vi "R30.vi"() -> ()   [LabVIEW 2016, in "beamline sections.lvlib" / "R30  library.lvlib"]
uses:
  R30/R30  library.lvlib
  save load/saveloadprev.ctl
  controls/Faraday cup states.ctl
  low energy end/Low energy end/Low energy end llb.lvlib
  Transmission/transmission.lvlib
  High energy end/High energy llb.lvlib
  save load/SaveLoad.lvlib
panel:
  in  "Tab Control":T1(tab)
  in  "Cluster 2":T2
  out "R30 steer +X":dbl
  out "R30 steer -X":dbl
  out "R30 steer +Y":dbl
  out "R30 steer -Y":dbl
  out "R30 steer +X Set":dbl
  out "R30 steer -X Set":dbl
  out "R30 steer +Y Set":dbl
  out "R30 steer -Y Set":dbl
  in  "stop":bool
  out "R30 Mag Y-steerer I read":dbl format="%#_3g"
  out "Mag Y-steerer range":bool=TRUE
  out "ESA range":bool=TRUE
  out "ESA V Read":dbl min=0.0 max=200.0
  in  "ESA":dbl(slide) min=0.0 max=60.0 scale=0.0..75.0
  in  "R30 Y steerer":dbl(slide) min=-10.0 max=10.0 scale=-10.0..10.0
  in  "R30 Quad A":dbl(slide) min=0.0 max=2.0 step=0.01 scale=0.0..2.0
  in  "R30 X steerer":dbl(slide) min=-10.0 max=10.0 scale=-10.0..10.0
  in  "R30 Quad B":dbl(slide) min=0.0 max=2.0 step=0.01 scale=0.0..2.0
  out "R30 Quad A I read":dbl min=0.0 max=200.0 format="%#_3g"
  out "R30 Quad B I read":dbl min=0.0 max=200.0 format="%#_3g"
  out "R30 quad Range":bool=TRUE
  out "R30 Steerer X Read":dbl format="%#_5g"
  out "R30 Steerer Y Read":dbl format="%#_4g"
  out "R30 Steerer range":bool=TRUE
  in  "Mag Y steerer":dbl(slide) min=-3.0 max=3.0 scale=-3.0..3.0
  out "R30 Mag Y-steerer V read":dbl
  out "R30 Detector FC status":T3
  in  "R30 temp file":path=path "D:/Main Tune Parameters/Temp Configs/R30.txt"
  out "SV error":errorcluster
  out "SaveLoad error":errorcluster
  out "R30-1-RT Error":errorcluster
  out "R30-1-FPGA Error":errorcluster
  # "R30"
  # "R30 Steerer Plate Voltages"
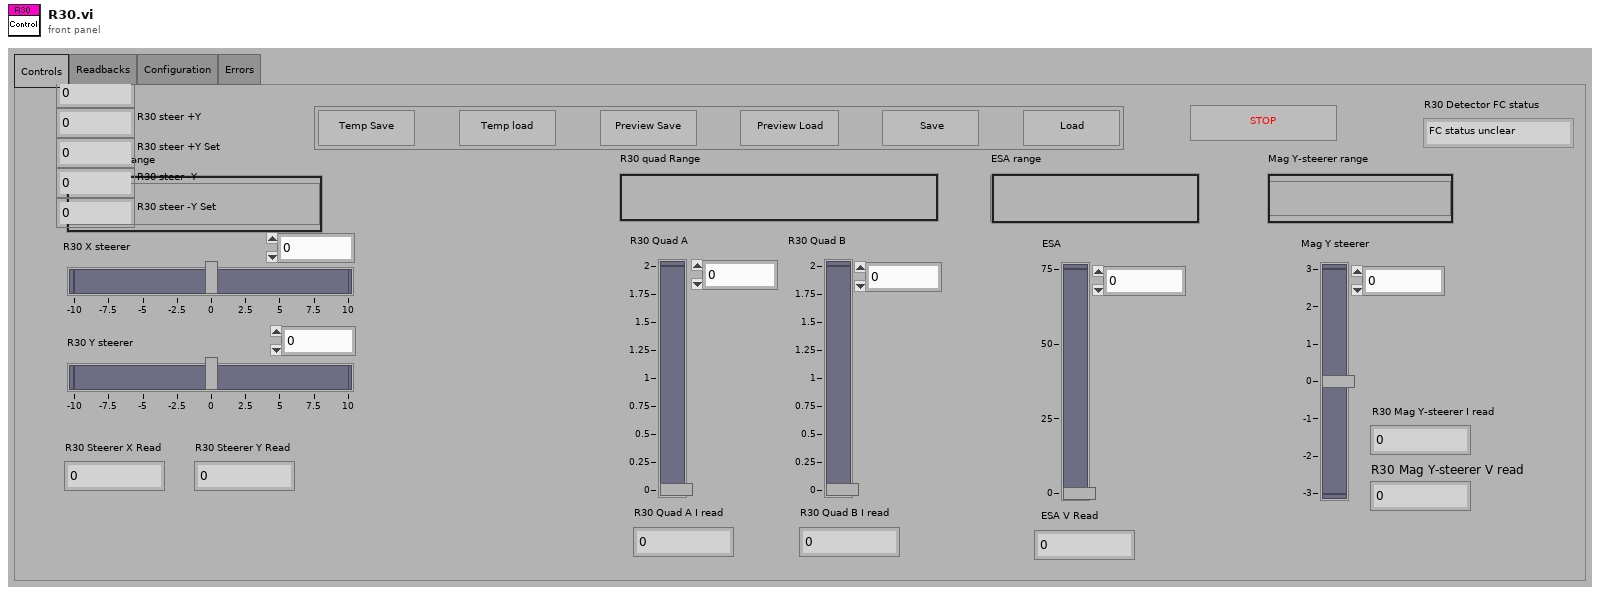
[diagram p1: front panel]
types:
  T1 = enum32{"Controls", "Readbacks", "Configuration", "Errors"}
  T2 = typedef "saveloadprev.ctl" = cluster{"Temp Save":bool, "Temp Load":bool, "Save":bool, "Load":bool, "Preview Save":bool, "Preview Load":bool}
  T3 = typedef "Faraday cup states.ctl" = enum16{"FC status unclear", "FC in", "FC out"}
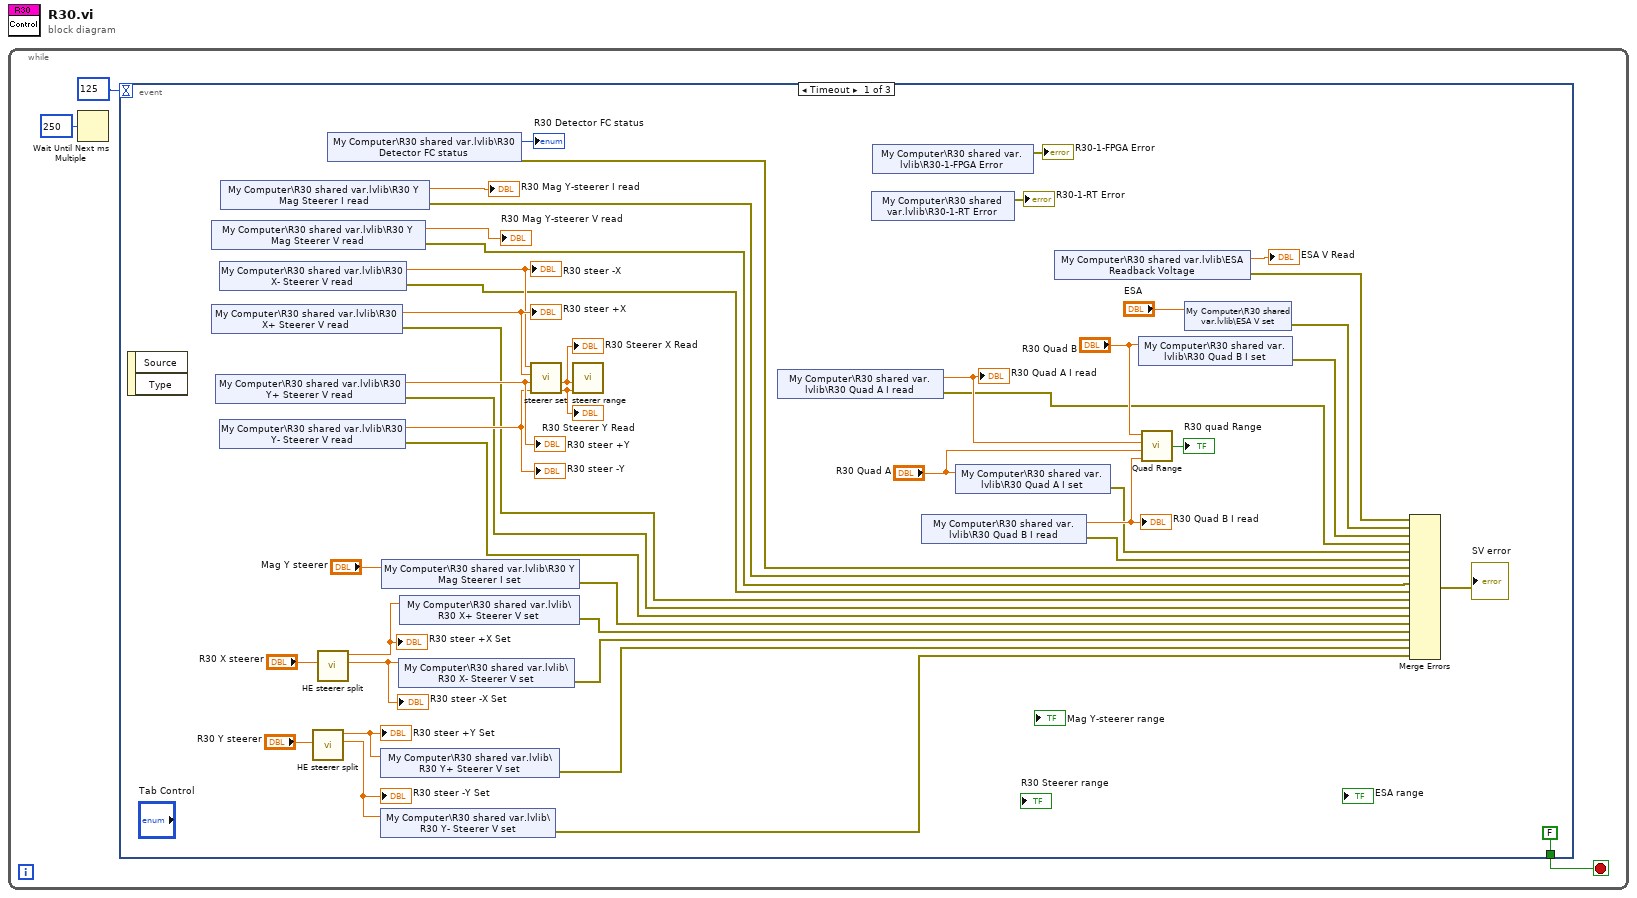
[diagram p0: block diagram]
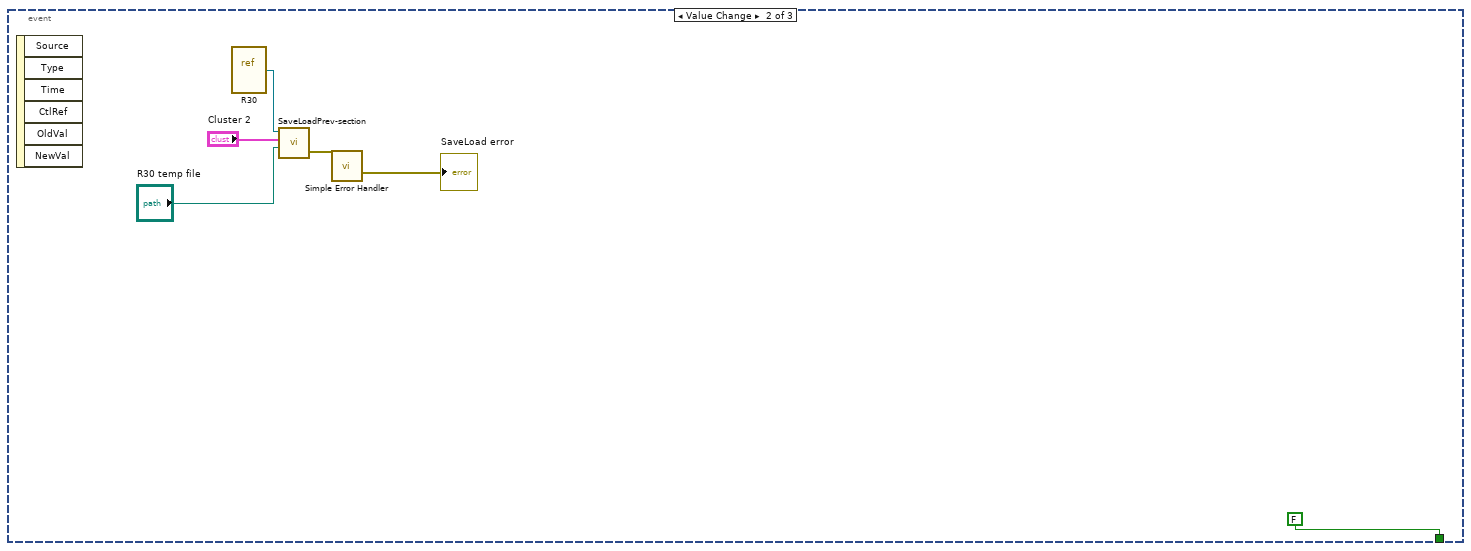
[diagram p2: hidden frame]
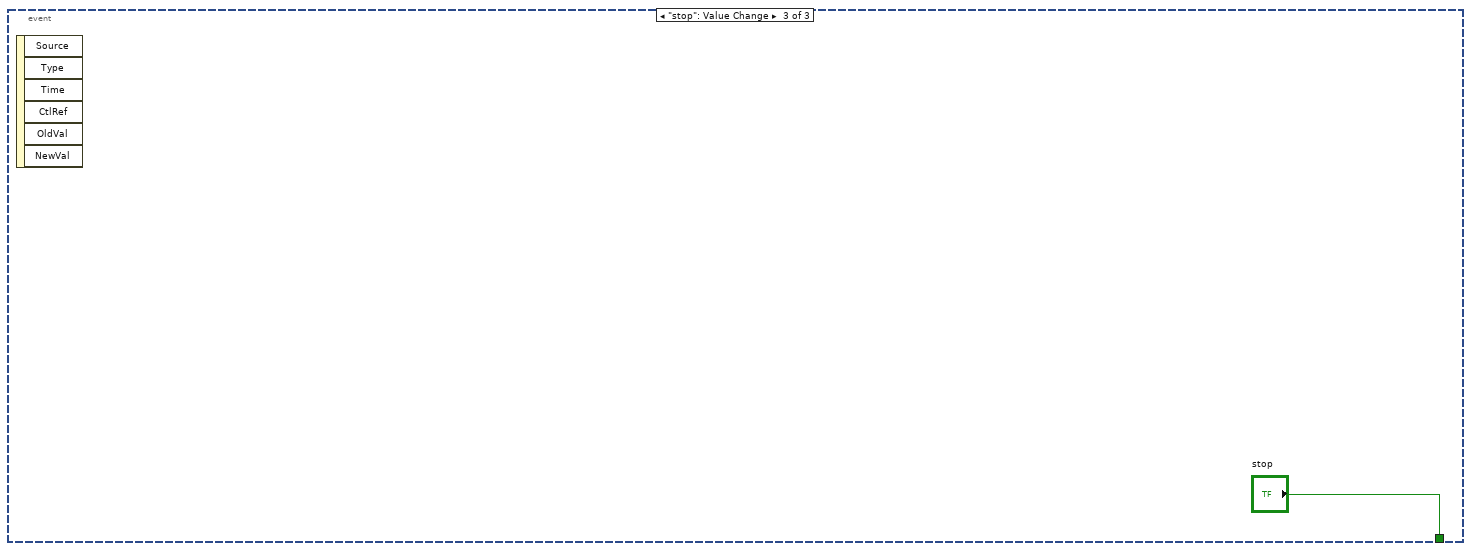
[diagram p3: hidden frame]
diagram:
  n1 = while {
    stop <- w1 stop-if-true
    n2 = Wait Until Next ms Multiple(millisecond multiple=u32 250) -> ()  [unwired: 1 out]
    n3 = event shown="[0] Timeout" {
      selector: _ -> [_ _ _]
      dyn-events: _ -> [_ _ _]
      timeout: 125 -> [_ _ _]
      tunnel: [FALSE ("stop") FALSE ("stop") "stop"] -> w1
      event Timeout {
        n4 = event-data() -> ()  [unwired: 1 in, 2 out]
        n5 = shared-variable "My Computer\\R30 shared var.lvlib\\R30 Y Mag Steerer V read"() -> (→"R30 Mag Y-steerer V read":dbl, error out=w6:errorcluster)  [unwired: 1 in]
        n6 = shared-variable "My Computer\\R30 shared var.lvlib\\R30 X+ Steerer V read"() -> (w43:dbl, error out=w20:errorcluster)  [unwired: 1 in]
        "R30 steer +X" <- w43
        n7 = shared-variable "My Computer\\R30 shared var.lvlib\\R30 Y+ Steerer V read"() -> (w47:dbl, error out=w21:errorcluster)  [unwired: 1 in]
        "R30 steer +Y" <- w47
        n8 = shared-variable "My Computer\\R30 shared var.lvlib\\R30 X- Steerer V read"() -> (w42:dbl, error out=w19:errorcluster)  [unwired: 1 in]
        "R30 steer -X" <- w42
        n9 = shared-variable "My Computer\\R30 shared var.lvlib\\R30 Y- Steerer V read"() -> (w46:dbl, error out=w22:errorcluster)  [unwired: 1 in]
        "R30 steer -Y" <- w46
        n10 = shared-variable "My Computer\\R30 shared var.lvlib\\R30 Y Mag Steerer I read"() -> (→"R30 Mag Y-steerer I read":dbl, error out=w18:errorcluster)  [unwired: 1 in]
        n11 = call "HE steerer split.vi"("Steerer in"="R30 Y steerer") -> ("Steerer +"=w36:dbl, "Steerer -"=w41:dbl)  [unwired: 7 out]
        "R30 steer +Y Set" <- w36
        "R30 steer -Y Set" <- w41
        n12 = call "HE steerer split.vi"("Steerer in"="R30 X steerer") -> ("Steerer +"=w39:dbl, "Steerer -"=w40:dbl)  [unwired: 7 out]
        "R30 steer +X Set" <- w39
        "R30 steer -X Set" <- w40
        n13 = shared-variable "My Computer\\R30 shared var.lvlib\\R30 Detector FC status"() -> (→"R30 Detector FC status":T3, error out=w17:errorcluster)  [unwired: 1 in]
        n14 = shared-variable "My Computer\\R30 shared var.lvlib\\R30 Y+ Steerer V set"(w36) -> (error out=w25:errorcluster)  [unwired: 1 in]
        n15 = shared-variable "My Computer\\R30 shared var.lvlib\\R30 Y- Steerer V set"(w41) -> (error out=w26:errorcluster)  [unwired: 1 in]
        n16 = shared-variable "My Computer\\R30 shared var.lvlib\\R30 Y Mag Steerer I set"("Mag Y steerer") -> (error out=w8:errorcluster)  [unwired: 1 in]
        n17 = shared-variable "My Computer\\R30 shared var.lvlib\\R30 X- Steerer V set"(w40) -> (error out=w24:errorcluster)  [unwired: 1 in]
        n18 = shared-variable "My Computer\\R30 shared var.lvlib\\R30 X+ Steerer V set"(w39) -> (error out=w23:errorcluster)  [unwired: 1 in]
        n19 = call "steerer set.vi"("Injector image X  -"=w42, "Injector image X +"=w43, "Injector image Y  -"=w47, "Injector image Y +"=w46) -> ("Steerer X"=w44:dbl, "Steerer Y"=w45:dbl)  [unwired: 4 out]
        "R30 Steerer X Read" <- w44
        "R30 Steerer Y Read" <- w45
        n20 = call "steerer range.vi"("Steerer Y Voltage"=w45, "Steerer X Voltage"=w44) -> ()  [unwired: 2 in, 4 out]
        n21 = shared-variable "My Computer\\R30 shared var.lvlib\\R30 Quad A I read"() -> (w29:dbl, error out=w14:errorcluster)  [unwired: 1 in]
        "R30 Quad A I read" <- w29
        n22 = shared-variable "My Computer\\R30 shared var.lvlib\\R30-1-RT Error"() -> (→"R30-1-RT Error":errorcluster)  [unwired: 1 in, 1 out]
        n23 = shared-variable "My Computer\\R30 shared var.lvlib\\R30-1-FPGA Error"() -> (→"R30-1-FPGA Error":errorcluster)  [unwired: 1 in, 1 out]
        n24 = shared-variable "My Computer\\R30 shared var.lvlib\\R30 Quad B I read"() -> (w28:dbl, error out=w16:errorcluster)  [unwired: 1 in]
        "R30 Quad B I read" <- w28
        n25 = shared-variable "My Computer\\R30 shared var.lvlib\\R30 Quad A I set"("R30 Quad A") -> (error out=w15:errorcluster)  [unwired: 1 in]
        n26 = shared-variable "My Computer\\R30 shared var.lvlib\\ESA Readback Voltage"() -> (→"ESA V Read":dbl, error out=w11:errorcluster)  [unwired: 1 in]
        n27 = shared-variable "My Computer\\R30 shared var.lvlib\\R30 Quad B I set"("R30 Quad B") -> (error out=w13:errorcluster)  [unwired: 1 in]
        n28 = call "Quad Range.vi"("Transmission Quad B read"=w28, "Transmission Quad A set"="R30 Quad A", "Transmission Quad A read"=w29, "Transmission Quad B set"="R30 Quad B") -> ("Quad range?"=→"R30 quad Range":bool)
        n29 = shared-variable "My Computer\\R30 shared var.lvlib\\ESA V set"("ESA") -> (error out=w12:errorcluster)  [unwired: 1 in]
        n30 = Merge Errors(w11, w12, w13, w14, w15, w16, w17, w18, w6, w19, w20, w21, w22, w8, w23, w24, w25, w26) -> (→"SV error":errorcluster)
      }
      event Value Change {
        n31 = event-data() -> ()  [unwired: 1 in, 6 out]
        n32 = vi-ref "R30.vi"() -> (w50:refnum<vi>)
        n33 = call "SaveLoadPrev-section.vi"("file path (use dialog)"="R30 temp file", "Cluster 2"="Cluster 2", "VI Refnum"=w50) -> ("error out"=w52:errorcluster)  [unwired: 2 in]
        n34 = call <vilib>:"Simple Error Handler.vi"("error in (no error)"=w52) -> ("error out"=→"SaveLoad error":errorcluster)  [unwired: 4 in, 4 out]
      }
      event "stop": Value Change {
        n35 = event-data() -> ()  [unwired: 1 in, 6 out]
      }
    }
  }
